vi "Initialize.vi"(8 "error in":errorcluster, 10 "parameters":variant, 11 "Abstract Engine in":refnum<class "Abstract Engine.lvclass">) -> (0 "error out":errorcluster, 2 "summary":T2[](array[typedef]), 3 "data value reference":T1)   [LabVIEW 2025, in "Abstract Engine.lvlib" / "Abstract Engine.lvclass"]
doc: "Initializes the data of a node to its default state.\nThe object is not created inside of this VI, because it is created from a File depending on user selection.\nCopyright 2017 National Instruments Corporation\n\nLicensed under the Apache License, Version 2.0 (the \"License\"); you may not use this file except in compliance with the License. You may obtain a copy of the License at http://www.apache.org/licenses/LICENSE-2.0\nUnless required by applicable law or agreed to in writing, software distributed under the License is distributed on an \"AS IS\" BASIS, WITHOUT WARRANTIES OR CONDITIONS OF ANY KIND, either express or implied. See the License for the specific language governing permissions and limitations under the License."
uses:
  Abstract Engine.lvclass
  Users/Public/Documents/Sandia National Labs/TSS Plugin/CEF.lvlibp/Node/Summary.ctl
  Users/Public/Documents/Sandia National Labs/TSS Plugin/CEF.lvlibp/Node/NodeRef.ctl
  Users/Public/Documents/Sandia National Labs/TSS Plugin/CEF.lvlibp/Node/CEF_Node.lvclass
  Abstract Engine.lvclass/Abstract Engine.ctl
  <vilib>/Utility/sysdir.llb/System Directory Type.ctl
  Engine configuration/Engine configuration.lvclass/Engine configuration.ctl
  <vilib>/Utility/error.llb/Trim Whitespace One-Sided.vi
  Users/Public/Documents/Sandia National Labs/TSS Plugin/CEF.lvlibp/serializable node/CEF_serializable node.lvclass
  Engine configuration/Engine configuration.lvclass
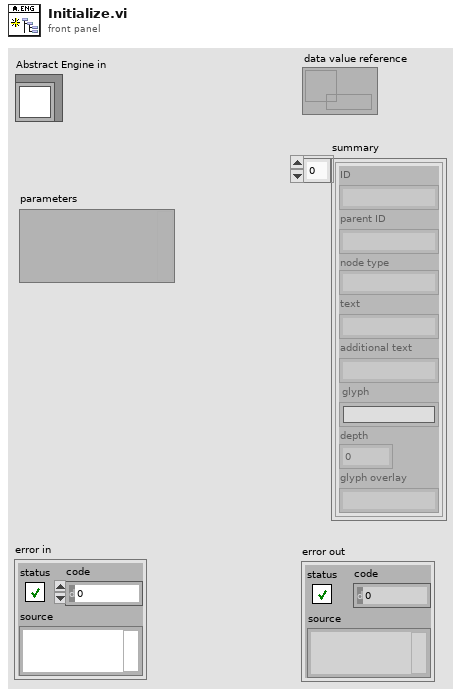
[diagram p1: front panel]
types:
  T1 = typedef "CEF.lvlibp/CEF_Node.lvclass/NodeRef.ctl" = refnum<data-value>
  T2 = typedef "CEF.lvlibp/CEF_Node.lvclass/Summary.ctl" = cluster{"ID":string, "parent ID":string, "node type":string, "text":string, "additional text":string, "glyph":string, "depth":i32, "glyph overlay":string}
  T3 = typedef "System Directory Type.ctl" = i32
  T4 = typedef "Abstract Engine.lvlib/Engine configuration.lvclass/Engine Setting.ctl" = cluster{"Enabled":bool, "IP Address":string, "Port":i32, "Description":string, "Type":string, "Version":string}
  T5 = cluster{"ID":string, "parent ID":string, "node type":string, "text":string, "additional text":string, "glyph":string, "depth":i32, "glyph overlay":string}[]
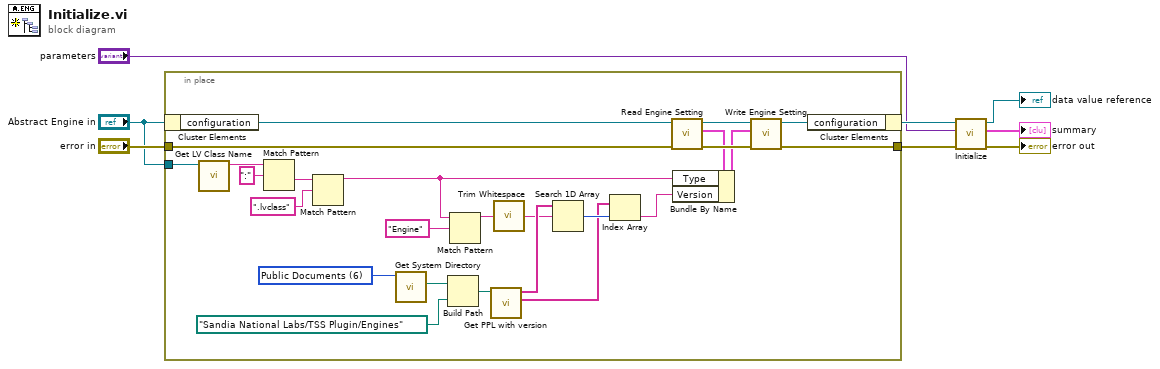
[diagram p0: block diagram]
diagram:
  n1 = in-place {
    in-place-border: [w33] -> w5
    in-place-border: "error in" -> [w21]
    in-place-border: "Abstract Engine in" -> [w26]
    w18 = T3 6 items=["User Home"=0, "User Desktop"=1, "User Documents"=2, "User Application Data"=3, "User Preferences"=4, "User Temporary"=5, "Public Documents"=6, "Public Application Data"=7, "Public Preferences"=8, "Public Cache"=13, "System Core Libraries"=9, "System Installed Libraries"=10, "Application Files"=11, "Boot Volume Root"=12] ("system directory type")
    n2 = in-place-cluster #1("Abstract Engine in") -> ("configuration"=w31:refnum<class "Engine configuration.lvclass">)
    n3 = call <vilib>:"Get LV Class Name.vi"("object"=w26) -> ("class name"=w22:string)  [unwired: 9 in, 1 out]
    n4 = Match Pattern(string=w22, regular expression=":") -> (after substring=w27:string)  [unwired: 1 in, 3 out]
    n5 = Match Pattern(string=w27, regular expression=".lvclass") -> (before substring=w11:string)  [unwired: 1 in, 3 out]
    n6 = call <vilib>:"Get System Directory.vi"("system directory type"=w18) -> ("system directory"=w19:path)  [unwired: 10 in]
    n7 = Build Path(base path=w19, name or relative path=path "Sandia National Labs/TSS Plugin/Engines" ("PPL folder")) -> (appended path=w20:path)
    n8 = Match Pattern(string=w11, regular expression="Engine") -> (before substring=w10:string)  [unwired: 1 in, 3 out]
    n9 = call "Get PPL with version.vi"("Plugin path"=w20) -> ("Plugin"=w13:string[], "Version"=w16:string[])  [unwired: 9 in]
    n10 = call <vilib>:"Trim Whitespace.vi"("string"=w10) -> ("trimmed string"=w9:string)  [unwired: 1 in]
    n11 = Search 1D Array(1D array=w16, element=w9) -> (index of element=w15:i32)  [unwired: 1 in]
    n12 = Index Array(array=w13, index=w15) -> (element=w14:string)
    n13 = call "Read Engine Setting.vi"("error in (no error)"=w21, "Engine configuration in"=w31) -> ("error out"=w32:errorcluster, "Engine Setting"=w29:T4, "Engine configuration out"=w30:refnum<class "Engine configuration.lvclass">)  [unwired: 7 in]
    n14 = Bundle By Name(cluster=w29, "Type"=w11, "Version"=w14) -> (w28:T4)
    n15 = call "Write Engine Setting.vi"("error in (no error)"=w32, "Engine Setting"=w28, "Engine configuration in"=w30) -> ("error out"=w33:errorcluster, "Engine configuration out"=w23:refnum<class "Engine configuration.lvclass">)  [unwired: 7 in]
    n16 = in-place-cluster #1("configuration"=w23) -> (w2:refnum<class "Abstract Engine.lvclass">)
  }
  n17 = call-parent "Initialize.vi"("error in"=w5, "parameters"="parameters", "CEF_Serialize node in"=w2) -> ("error out"=→"error out":errorcluster, "summary"=→"summary":T5, "data value reference"=→"data value reference":refnum<data-value>)  [unwired: 6 in]
